vi "PDE_Sensor_Read.vi"(8 "Error In":errorcluster, 9 "Pressure Freq":dbl, 10 "Temperature Freq":dbl, 11 "Sampling Time":dbl=1.0) -> (0 "Error Out":errorcluster, 1 "Pressure Data":waveform(dbl)[](array[waveform]), 2 "Temperature Data":waveform(dbl)[](array[waveform]))   [LabVIEW 2016]
uses:
  <vilib>/DAQmx/read.llb/DAQmx Read (Analog 1D Wfm NChan NSamp).vi
  <vilib>/DAQmx/create/channels.llb/DAQmx Create Channel (AI-Temperature-Thermocouple).vi
  <resource>/objmgr/daqmx.rc
  <vilib>/DAQmx/configure/timing.llb/DAQmx Timing (Sample Clock).vi
  <vilib>/DAQmx/create/channels.llb/DAQmx Create Channel (AI-Current-Basic).vi
  <vilib>/DAQmx/create/channels.llb/DAQmx Create Channel (AI-Voltage-Basic).vi
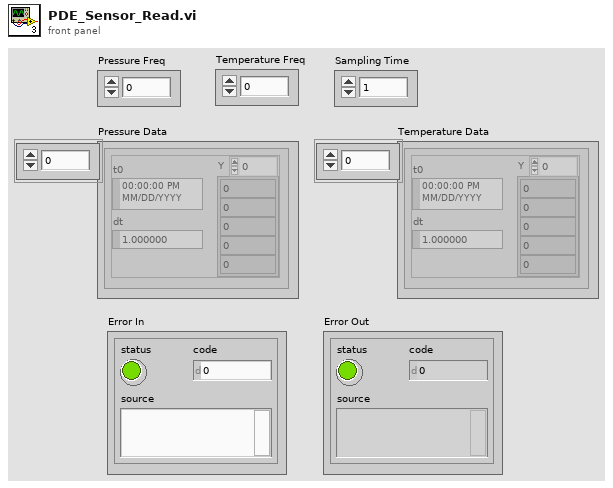
[diagram p1: front panel]
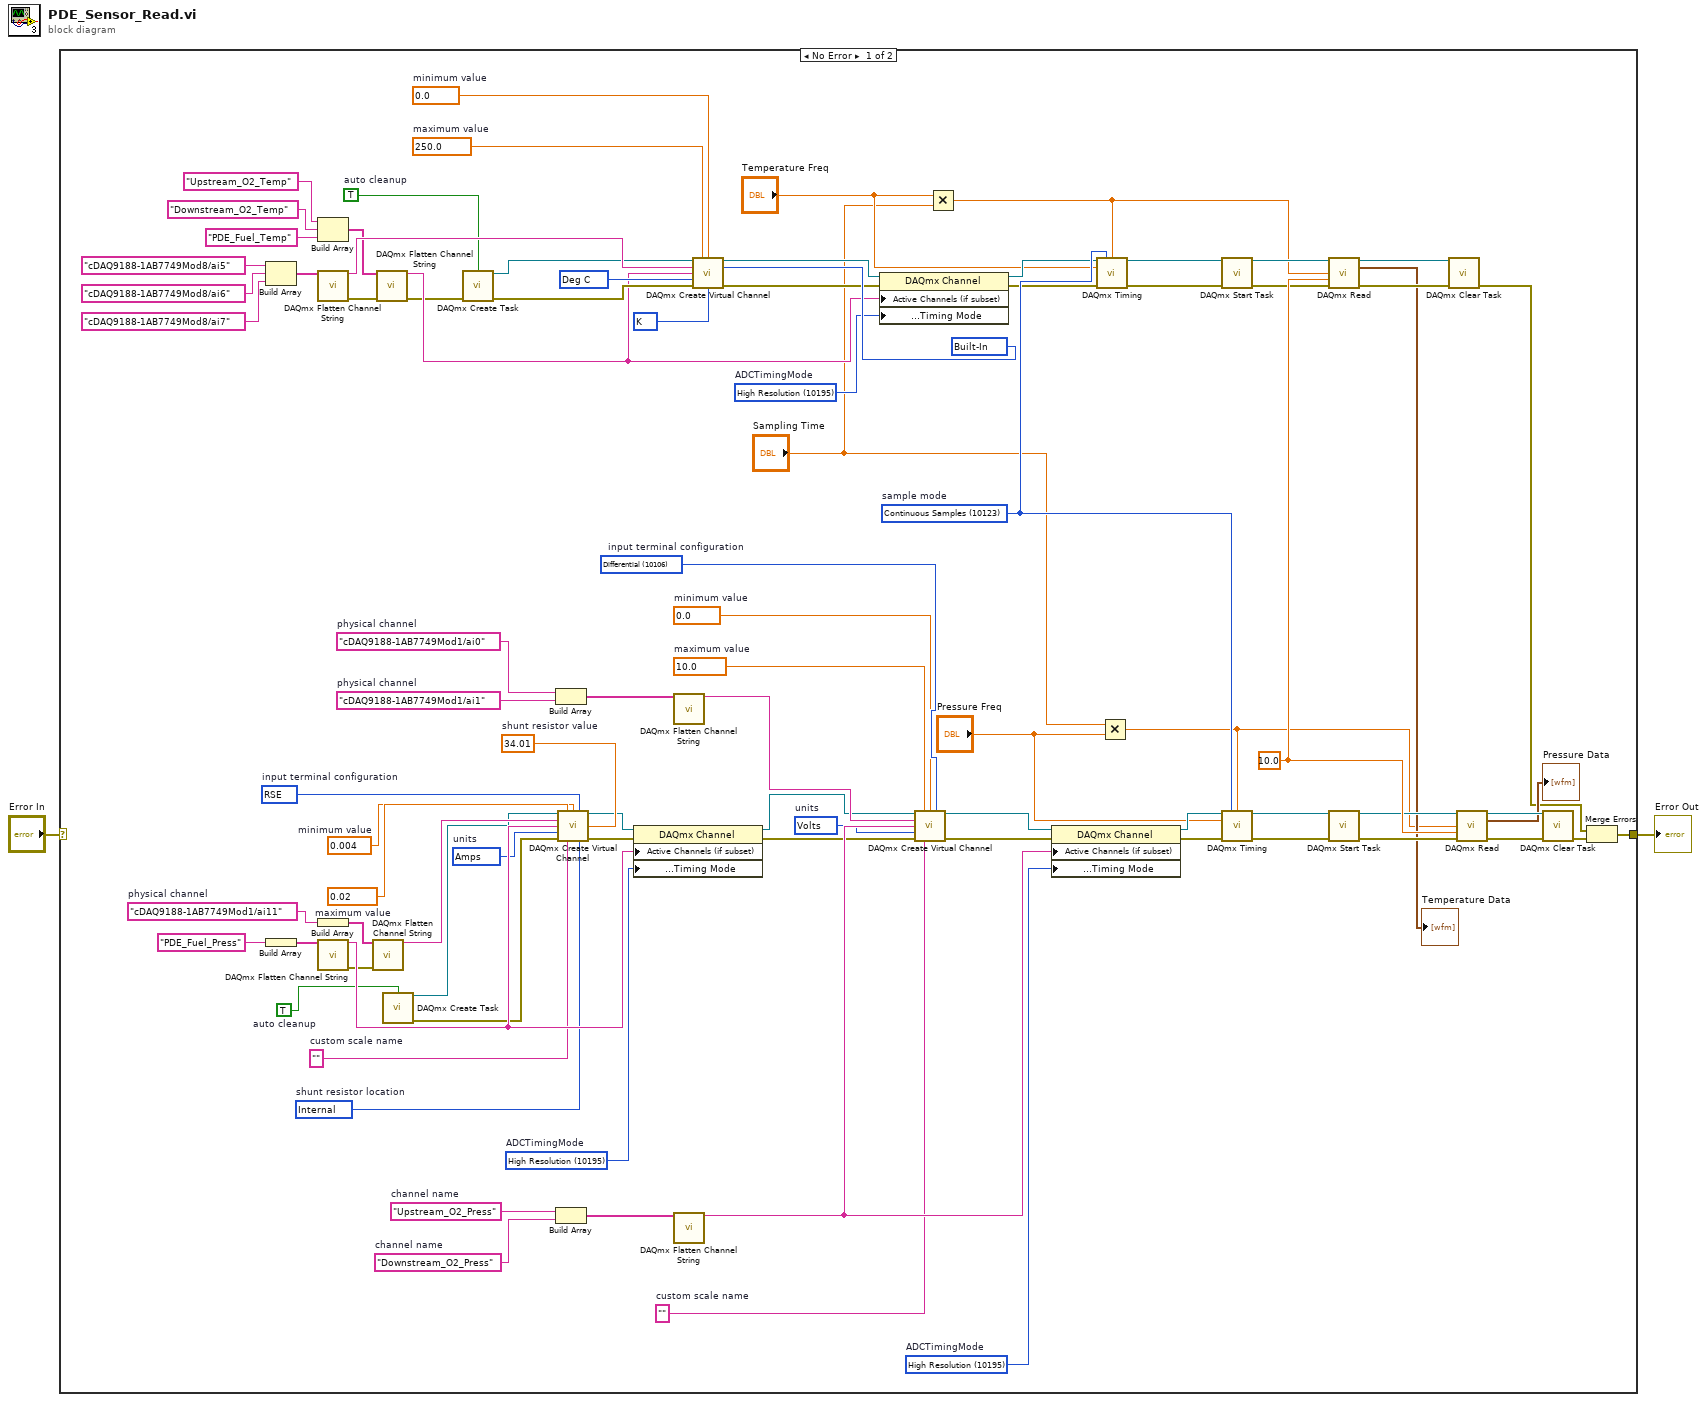
[diagram p0: block diagram]
diagram:
  n1 = case shown="No Error" "Error In" {
    selector: "Error In" -> [_ w92]
    tunnel: [w3 w92] -> w1
    frame No Error {
      w80 = 10.0 ("timeout")
      w74 = 10195 items=["High Resolution"=10195, "High Speed"=14712, "Best 50 Hz Rejection"=14713, "Best 60 Hz Rejection"=14714]  # ADCTimingMode
      w86 = "Downstream_O2_Press"  # channel name
      w83 = "cDAQ9188-1AB7749Mod1/ai1"  # physical channel
      w73 = 10106 items=["default"=-1, "RSE"=10083, "NRSE"=10078, "Differential"=10106, "Pseudodifferential"=12529]  # input terminal configuration
      w88 = 10348 items=["Volts"=10348, "From Custom Scale"=10065]  # units
      w87 = "Upstream_O2_Press"  # channel name
      w72 = ""  # custom scale name
      w71 = 0.0  # minimum value
      w70 = 10.0  # maximum value
      w82 = "cDAQ9188-1AB7749Mod1/ai0"  # physical channel
      w68 = "cDAQ9188-1AB7749Mod1/ai11"  # physical channel
      w75 = 10123 items=["Finite Samples"=10178, "Continuous Samples"=10123, "Hardware Timed Single Point"=12522]  # sample mode
      w47 = 10195 items=["High Resolution"=10195, "High Speed"=14712, "Best 50 Hz Rejection"=14713, "Best 60 Hz Rejection"=14714]  # ADCTimingMode
      w48 = 10083 items=["default"=-1, "RSE"=10083, "NRSE"=10078, "Differential"=10106, "Pseudodifferential"=12529]  # input terminal configuration
      w49 = 10342 items=["Amps"=10342, "From Custom Scale"=10065]  # units
      w50 = 34.01  # shunt resistor value
      w51 = 10200 items=["Internal"=10200, "External"=10167]  # shunt resistor location
      w53 = ""  # custom scale name
      w54 = 0.004  # minimum value
      w55 = 0.02  # maximum value
      w57 = TRUE  # auto cleanup
      w42 = 10143 items=["Deg C"=10143, "Deg F"=10144, "Kelvins"=10325, "Deg R"=10145, "From Custom Scale"=10065] ("units")
      w41 = 10073 items=["J"=10072, "K"=10073, "N"=10077, "R"=10082, "S"=10085, "T"=10086, "B"=10047, "E"=10055] ("thermocouple type")
      w40 = 10200 items=["Built-In"=10200, "Constant Value"=10116, "Channel"=10113] ("cjc source")
      w31 = 10195 items=["High Resolution"=10195, "High Speed"=14712, "Best 50 Hz Rejection"=14713, "Best 60 Hz Rejection"=14714]  # ADCTimingMode
      w34 = 0.0  # minimum value
      w35 = 250.0  # maximum value
      w37 = TRUE  # auto cleanup
      n2 = Build Array("cDAQ9188-1AB7749Mod8/ai5" ("element"), "cDAQ9188-1AB7749Mod8/ai6" ("element"), "cDAQ9188-1AB7749Mod8/ai7" ("element")) -> (w43:string[])
      n3 = Build Array("PDE_Fuel_Press" ("element")) -> (w60:string[])
      n4 = Build Array("Upstream_O2_Temp" ("name to assign"), "Downstream_O2_Temp" ("name to assign"), "PDE_Fuel_Temp" ("name to assign")) -> (w20:string[])
      n5 = call <vilib>:"DAQmx Flatten Channel String.vi"("names in"=w43) -> ("names out"=w39:string, "error out"=w4:errorcluster)  [unwired: 13 in]
      n6 = Build Array(w68) -> (w62:string[])
      n7 = call <vilib>:"DAQmx Flatten Channel String.vi"("names in"=w60) -> ("names out"=w61:string, "error out"=w5:errorcluster)  [unwired: 13 in]
      n8 = call <vilib>:"DAQmx Flatten Channel String.vi"("names in"=w62, "error in"=w5) -> ("names out"=w59:string)  [unwired: 12 in, 1 out]
      n9 = call <vilib>:"DAQmx Flatten Channel String.vi"("names in"=w20, "error in"=w4) -> ("names out"=w16:string, "error out"=w15:errorcluster)  [unwired: 12 in]
      n10 = call <vilib>:"DAQmx Create Task.vi"("auto cleanup"=w57) -> ("task out"=w56:refnum<k21>, "error out"=w58:errorcluster)  [unwired: 4 in, 9 out]
      n11 = call <vilib>:"DAQmx Create Task.vi"("auto cleanup"=w37, "error in"=w15) -> ("task out"=w36:refnum<k21>, "error out"=w38:errorcluster)  [unwired: 3 in, 9 out]
      n12 = Build Array(w82, w83) -> (w81:string[])
      n13 = Build Array(w87, w86) -> (w85:string[])
      n14 = call-poly <vilib>:"DAQmx Create Virtual Channel.vi"("task in"=w56, "maximum value"=w55, "minimum value"=w54, "input terminal configuration"=w48, "physical channels"=w59, "name to assign"=w61, "external shunt resistor value"=w50, "units"=w49, "error in"=w58, "custom scale name"=w53, "shunt resistor location"=w51) -> ("task out"=w46:refnum<k21>, "error out"=w52:errorcluster)  [unwired: 3 out]
      n15 = property class="DAQmx Channel"(reference=w46, error in=w52, "Active Channels (if subset)"=w61, "Analog Input:General Properties:Digitizer/ADC:Timing Mode"=w47) -> (reference out=w77:refnum<k21>, error out=w78:errorcluster)
      n16 = call <vilib>:"DAQmx Flatten Channel String.vi"("names in"=w81) -> ("names out"=w84:string)  [unwired: 13 in, 1 out]
      n17 = call <vilib>:"DAQmx Flatten Channel String.vi"("names in"=w85) -> ("names out"=w91:string)  [unwired: 13 in, 1 out]
      n18 = call-poly <vilib>:"DAQmx Create Virtual Channel.vi"("task in"=w36, "maximum value"=w35, "minimum value"=w34, "physical channels"=w39, "cjc source"=w40, "name to assign"=w16, "units"=w42, "error in"=w38, "thermocouple type"=w41) -> ("task out"=w30:refnum<k21>, "error out"=w33:errorcluster)  [unwired: 5 in]
      n19 = property class="DAQmx Channel"(reference=w30, error in=w33, "Active Channels (if subset)"=w16, "Analog Input:General Properties:Digitizer/ADC:Timing Mode"=w31) -> (reference out=w29:refnum<k21>, error out=w32:errorcluster)
      n20 = call-poly <vilib>:"DAQmx Create Virtual Channel.vi"("task in"=w77, "maximum value"=w70, "minimum value"=w71, "input terminal configuration"=w73, "physical channels"=w84, "name to assign"=w91, "units"=w88, "error in"=w78, "custom scale name"=w72) -> ("task out"=w89:refnum<k21>, "error out"=w90:errorcluster)  [unwired: 5 in]
      n21 = Multiply(x="Temperature Freq", y="Sampling Time") -> (x*y=w8:dbl)
      n22 = property class="DAQmx Channel"(reference=w89, error in=w90, "Active Channels (if subset)"=w91, "Analog Input:General Properties:Digitizer/ADC:Timing Mode"=w74) -> (reference out=w76:refnum<k21>, error out=w79:errorcluster)
      n23 = call-poly <vilib>:"DAQmx Timing.vi"("task/channels in"=w29, "sample mode"=w75, "samples per channel"=w8, "rate"="Temperature Freq", "error in"=w32) -> ("task out"=w44:refnum<k21>, "error out"=w45:errorcluster)  [unwired: 2 in, 7 out]
      n24 = Multiply(x="Sampling Time", y="Pressure Freq") -> (x*y=w7:dbl)
      n25 = call <vilib>:"DAQmx Start Task.vi"("task/channels in"=w44, "error in"=w45) -> ("task out"=w25:refnum<k21>, "error out"=w26:errorcluster)  [unwired: 12 out]
      n26 = call-poly <vilib>:"DAQmx Timing.vi"("task/channels in"=w76, "sample mode"=w75, "samples per channel"=w7, "rate"="Pressure Freq", "error in"=w79) -> ("task out"=w64:refnum<k21>, "error out"=w63:errorcluster)  [unwired: 2 in, 7 out]
      n27 = call-poly <vilib>:"DAQmx Read.vi"("task/channels in"=w25, "number of samples per channel"=w8, "timeout"=w80, "error in"=w26) -> ("task out"=w28:refnum<k21>, "data"=→"Temperature Data":waveform(dbl)[], "error out"=w27:errorcluster)  [unwired: 9 out]
      n28 = call <vilib>:"DAQmx Start Task.vi"("task/channels in"=w64, "error in"=w63) -> ("task out"=w21:refnum<k21>, "error out"=w22:errorcluster)  [unwired: 12 out]
      n29 = call <vilib>:"DAQmx Clear Task.vi"("task in"=w28, "error in"=w27) -> ("error out"=w11:errorcluster)  [unwired: 13 out]
      n30 = call-poly <vilib>:"DAQmx Read.vi"("task/channels in"=w21, "number of samples per channel"=w7, "timeout"=w80, "error in"=w22) -> ("task out"=w24:refnum<k21>, "data"=→"Pressure Data":waveform(dbl)[], "error out"=w23:errorcluster)  [unwired: 9 out]
      n31 = call <vilib>:"DAQmx Clear Task.vi"("task in"=w24, "error in"=w23) -> ("error out"=w12:errorcluster)  [unwired: 13 out]
      n32 = Merge Errors(w11, w12) -> (w3:errorcluster)
    }
    frame Error {
    }
  }
  "Error Out" <- w1
